vi "CSQ_Check.vi"(10 "y":u8=22, 11 "CSQ":u8[](array[numeric])=[16, 25, 32, 33, 34, 255]) -> (2 "P/F":bool, 3 "Fail count":string)   [LabVIEW 2024, in "Test_2.lvlib"]
uses:
  Test_2.lvlib
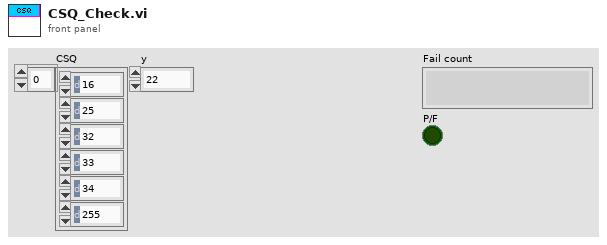
[diagram p1: front panel]
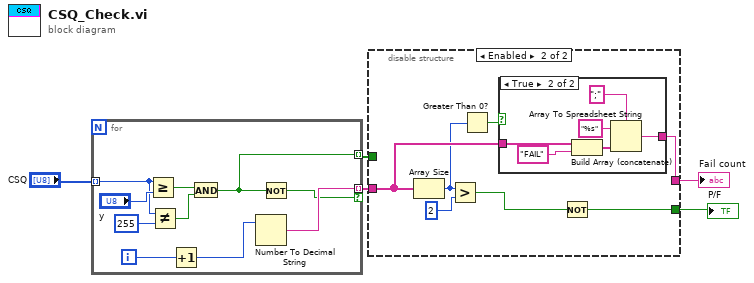
[diagram p0: block diagram]
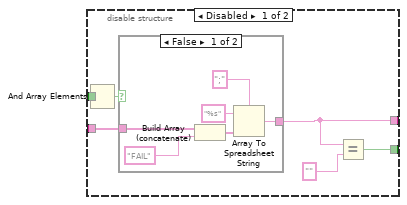
[diagram p2: hidden frame]
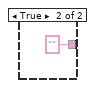
[diagram p3: hidden frame]
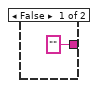
[diagram p4: hidden frame]
diagram:
  n1 = for {
    tunnel: "CSQ" -> [w12] mode=indexing
    tunnel: [w7] -> w4 mode=indexing
    tunnel: [w8] -> w3 mode=indexing if=w6
    i -> [w10]
    n2 = Greater Or Equal?(x=w12, y="y") -> (x >= y?=w14:bool)
    n3 = Not Equal?(x=w12, y=u8 255) -> (x != y?=w13:bool)
    n4 = Increment(x=w10) -> (x+1=w9:i32)
    n5 = And(x=w14, y=w13) -> (x .and. y?=w7:bool)
    n6 = Number To Decimal String(number=w9) -> (decimal integer string=w8:string)  [unwired: 1 in]
    n7 = Not(x=w7) -> (.not. x?=w6:bool)
  }
  n8 = disable-structure shown="Enabled" {
    disable-tunnel: w4 -> [w21 _]
    disable-tunnel: w3 -> [w19 w33]
    disable-tunnel: [w17 w32] -> w2
    disable-tunnel: [w16 w34] -> w1
    frame Disabled {
      n9 = And Array Elements(Boolean array=w21) -> (logical AND=w20:bool)
      n10 = case shown="False" w20 {
        tunnel: w19 -> [w27 _]
        tunnel: [w22 ""] -> w17
        frame False {
          n11 = Build Array (concatenate)(w27, "FAIL") -> (w24:string[])
          n12 = Array To Spreadsheet String(delimiter (Tab)=";", array=w24, 3:"%s" ("format string")) -> (spreadsheet string=w22:string)
        }
        frame True {
        }
      }
      n13 = Equal?(x=w17, y="" ("spreadsheet string")) -> (x = y?=w16:bool)
    }
    frame Enabled {
      n14 = Array Size(array=w33) -> (size(s)=w29:i32)
      n15 = Greater?(x=w29, y=2) -> (0:w31:bool)
      n16 = Greater Than 0?(x=w29) -> (x > 0?=w30:bool)
      n17 = case shown="True" w30 {
        tunnel: w33 -> [_ w38]
        tunnel: ["" ("spreadsheet string") w37] -> w32
        frame False {
        }
        frame True {
          n18 = Build Array (concatenate)(w38, "FAIL") -> (w40:string[])
          n19 = Array To Spreadsheet String(delimiter (Tab)=";", array=w40, 3:"%s" ("format string")) -> (spreadsheet string=w37:string)
        }
      }
      n20 = Not(x=w31) -> (.not. x?=w34:bool)
    }
  }
  "Fail count" <- w2
  "P/F" <- w1
